vi "RT Main 7-7 - No FPGA (IMAQ).vi"() -> ()   [LabVIEW 2025]
doc: "The myRIO Custom FPGA Project template acquires button data from the onboard button and displays the button value on a Boolean indicator. The SYS.RDY indicator shows the FPGA status."
uses:
  SoC IP Library/Controls/Image Size.ctl
  <vilib>/userDefined/High Color/IMAQdx.ctl
  SoC IP Library/SoC IP Library.lvlib
  <vilib>/vision/driver/NI_Vision_Acquisition_Software.lvlib
  <vilib>/vision/NI_Vision_Development_Module.lvlib
panel:
  in  "Display?":bool
  out "Image Out":T1(plugin-control)
  out "Image In":T1(plugin-control)
  in  "Live":bool
  out "FPS":u32
  out "error out":errorcluster
  in  "Stop":bool
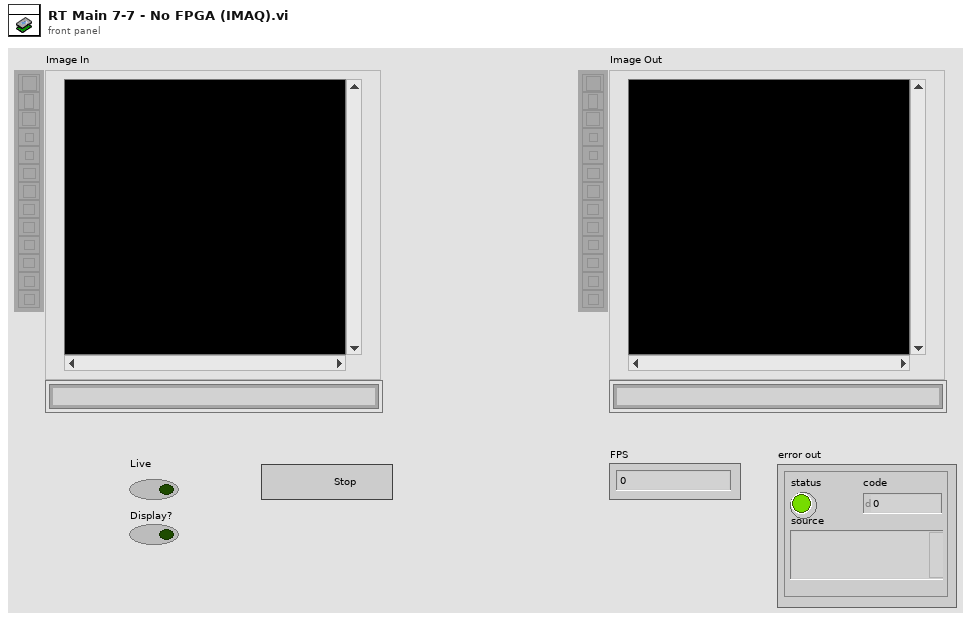
[diagram p1: front panel]
types:
  T1 = typedef "IMAQ Image.ctl" = refnum<image>
  T2 = typedef "IMAQdx.ctl" = refnum<k21>
  T3 = typedef "SoC IP Library.lvlib/Image Size.ctl" = cluster{"Rows (X)":u16, "Colums (Y)":u16}
  T4 = typedef "Image Type" = u32
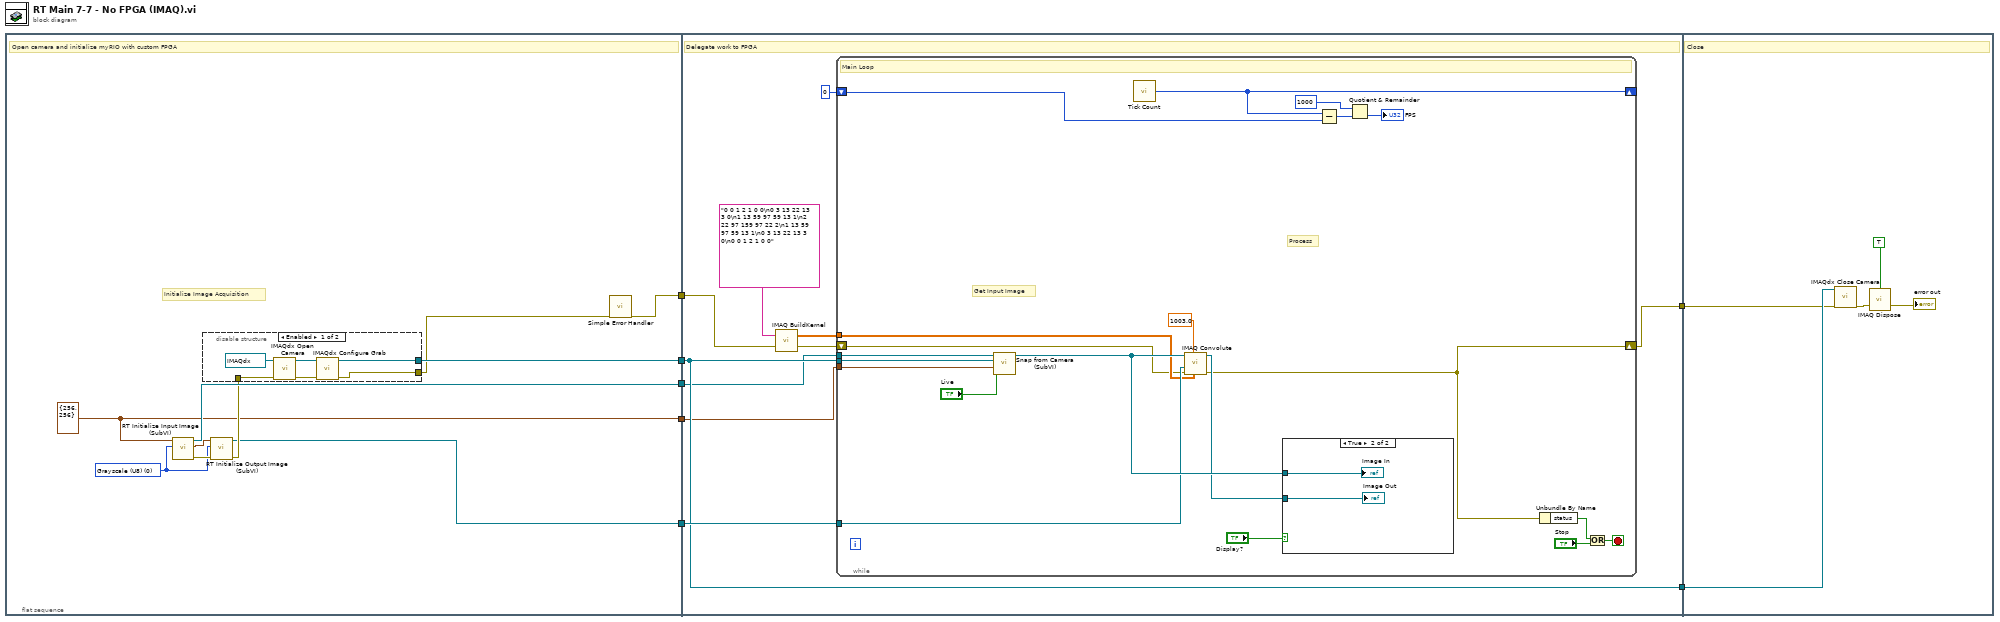
[diagram p0: block diagram]
diagram:
  n1 = flat-sequence {
    tunnel: [w12] -> w7
    tunnel: [w17] -> w6
    tunnel: [w16] -> w5
    tunnel: [w10] -> w4
    tunnel: [w9] -> w2
    tunnel: w7 -> [w33]
    tunnel: w6 -> [w32]
    tunnel: w5 -> [w31]
    tunnel: w4 -> [w29]
    tunnel: [w32] -> w3
    tunnel: w2 -> [w30]
    tunnel: [w25] -> w1
    tunnel: w3 -> [w58]
    tunnel: w1 -> [w57]
    frame #0 {
      w9 = T3 {"Rows (X)"=256, "Colums (Y)"=256} ("Image Size")
      w13 = T4 0 items=["Grayscale (U8)", "Grayscale (I16)", "Grayscale (SGL)", "Complex (CSG)", "RGB (U32)", "HSL (U32)", "RGB (U64)", "Grayscale (U16)"] ("Image Type")
      # "Initialize Image Acquisition"
      # "Open camera and initialize myRIO with custom FPGA"
      n2 = call "RT Initialize Input Image (SubVI).vi"("Image Type"=w13, "Image Size In"=w9) -> ("error out"=w15:errorcluster, "Input Image Size Out"=w11:T3, "Input Image Out"=w16:T1)  [unwired: 7 in]
      n3 = call "RT Initialize Output Image (SubVI).vi"("error in (no error)"=w15, "Image Type"=w13, "Image Size In"=w11) -> ("error out"=w14:errorcluster, "Output Image Out"=w12:T1)  [unwired: 7 in]
      n4 = disable-structure shown="Enabled" {
        disable-tunnel: [w20 _] -> w17
        disable-tunnel: w14 -> [w19 w24]
        disable-tunnel: [w18 w24] -> w8
        frame Enabled {
          n5 = call <vilib>:"IMAQdx Open Camera.vi"("error in"=w19, "Session In"=T2 "cam0") -> ("error out"=w22:errorcluster, "Session Out"=w21:T2)  [unwired: 8 in]
          n6 = call <vilib>:"IMAQdx Configure Grab.vi"("error in"=w22, "Session In"=w21) -> ("error out"=w18:errorcluster, "Session Out"=w20:T2)  [unwired: 8 in]
        }
        frame Disabled {
        }
      }
      n7 = call <vilib>:"Simple Error Handler.vi"("error in (no error)"=w8) -> ("error out"=w10:errorcluster)  [unwired: 4 in, 4 out]
    }
    frame #1 {
      # "Delegate work to FPGA"
      n8 = call "IMAQ BuildKernel"("Kernel String"="0 0 1 2 1 0 0\n0 3 13 22 13 3 0\n1 13 59 97 59 13 1\n2 22 97 159 97 22 2\n1 13 59 97 59 13 1\n0 3 13 22 13 3 0\n0 0 1 2 1 0 0", "error in (no error)"=w29) -> ("Kernel"=w27:sgl[][], "error out"=w26:errorcluster)  [unwired: 3 in]
      n9 = while {
        shift-right: [w52] -> _
        shift-left: u32 0 ("Tick Count(mSec)") -> [w51]
        tunnel: w32 -> [w50]
        tunnel: w33 -> [w40]
        tunnel: w31 -> [w49]
        tunnel: w30 -> [w46]
        tunnel: w27 -> [w39]
        shift-right: [w36] -> w25
        shift-left: w26 -> [w37]
        stop <- w53 stop-if-true
        # "Process"
        # "Get Input Image"
        # "Main Loop"
        n10 = call "Snap from Camera (SubVI).vi"("Live"="Live", "Image Size in"=w46, "Session In"=w50, "Image in"=w49) -> ("Image out"=w41:T1)  [unwired: 3 in, 4 out]
        n11 = call "Tick Count"() -> ("Tick Count(mSec)"=w52:u32)
        n12 = call "IMAQ Convolute"("Kernel"=w39, "Divider (kernel sum)"=sgl 1003.0, "error in (no error)"=w37, "Image Dst"=w40, "Image Src"=w41) -> ("error out"=w36:errorcluster, "Image Dst Out"=w38:T1)  [unwired: 5 in]
        n13 = case shown="True" "Display?" {
          tunnel: w41 -> [_ w56]
          tunnel: w38 -> [_ w55]
          frame False {
          }
          frame True {
            "Image In" <- w56
            "Image Out" <- w55
          }
        }
        n14 = Subtract(x=w52, y=w51) -> (x-y=w43:u32)
        n15 = Quotient & Remainder(x=u32 1000, y=w43) -> (floor(x/y)=→"FPS":u32)  [unwired: 1 out]
        n16 = Unbundle By Name(w36) -> ("status"=w45:bool)
        n17 = Or(x=w45, y="Stop") -> (x .or. y?=w53:bool)
      }
    }
    frame #2 {
      # "Close"
      n18 = call <vilib>:"IMAQdx Close Camera.vi"("error in"=w57, "Session In"=w58) -> ("error out"=w59:errorcluster)  [unwired: 9 in]
      n19 = call "IMAQ Dispose"("All Images? (No)"=TRUE, "error in (no error)"=w59) -> ("error out"=→"error out":errorcluster)  [unwired: 4 in]
    }
  }
